vi "Boolean value.vi"() -> ()   [LabVIEW 2018]
panel:
  out "String":string
  in  "Boolean":bool
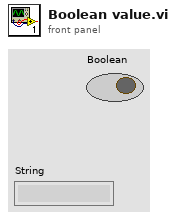
[diagram p1: front panel]
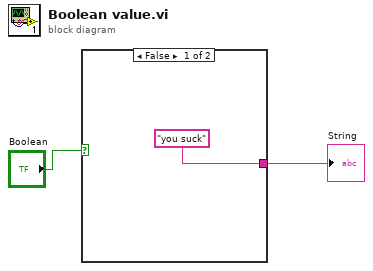
[diagram p0: block diagram]
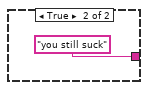
[diagram p2: hidden frame]
diagram:
  n1 = case shown="False" "Boolean" {
    tunnel: ["you suck" "you still suck"] -> w1
    frame False {
    }
    frame True {
    }
  }
  "String" <- w1
